vi "AllThingsBaxter_ROS.vi"   [LabVIEW 2012]
uses:
  <userlib>/ROSforLV/ROS/MessageBuilding/std_msgs/subs/boolScalar.vi
  <userlib>/ROSforLV/ROS/MessageBuilding/std_msgs/subs/durationScalar.vi
  <userlib>/ROSforLV/ROS/MessageBuilding/std_msgs/subs/float32Scalar.vi
  <userlib>/ROSforLV/ROS/MessageBuilding/std_msgs/subs/float64Scalar.vi
  <userlib>/ROSforLV/ROS/MessageBuilding/std_msgs/subs/i8Scalar.vi
  <userlib>/ROSforLV/ROS/MessageBuilding/std_msgs/subs/i16Scalar.vi
  <userlib>/ROSforLV/ROS/MessageBuilding/std_msgs/subs/i32Scalar.vi
  <userlib>/ROSforLV/ROS/MessageBuilding/std_msgs/subs/i64Scalar.vi
  <userlib>/ROSforLV/ROS/MessageBuilding/std_msgs/subs/stringScalar.vi
  <userlib>/ROSforLV/ROS/MessageBuilding/std_msgs/subs/timeScalar.vi
  <userlib>/ROSforLV/ROS/MessageBuilding/std_msgs/subs/u8Scalar.vi
  <userlib>/ROSforLV/ROS/MessageBuilding/std_msgs/subs/u16Scalar.vi
  <userlib>/ROSforLV/ROS/MessageBuilding/std_msgs/subs/u32Scalar.vi
  <userlib>/ROSforLV/ROS/MessageBuilding/std_msgs/subs/u64Scalar.vi
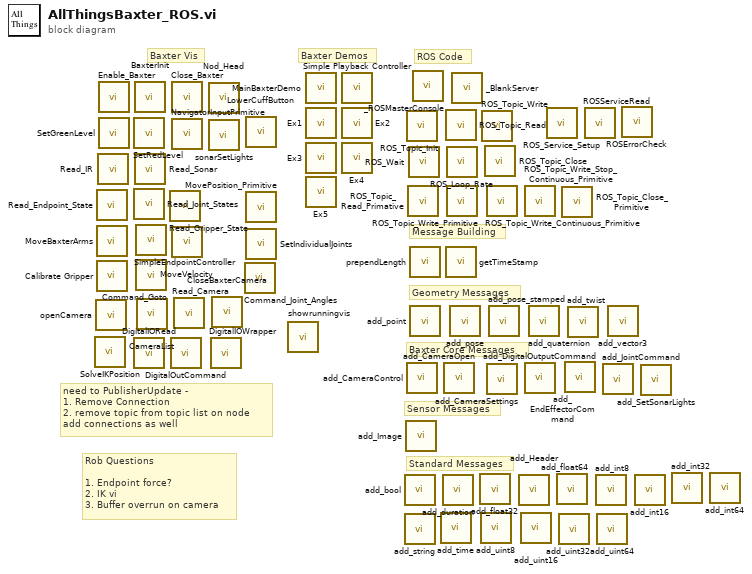
[diagram p0: block diagram]
diagram:
  # "Standard Messages"
  # "Sensor Messages"
  # "Baxter Core Messages"
  # "Geometry Messages"
  # "Message Building"
  # "Rob Questions\n\n1. Endpoint force?\n2. IK vi\n3. Buffer overrun on camera"
  # "need to PublisherUpdate - \n1. Remove Connection\n2. remove topic from topic list on node\nadd connections as well"
  # "ROS Code"
  # "Baxter Demos"
  # "Baxter Vis"
  n1 = call <userlib>:"SolveIKPosition.vi"() -> ()  [unwired: 7 in, 1 out]
  n2 = call <userlib>:"openCamera.vi"() -> ()  [unwired: 3 in, 2 out]
  n3 = call <userlib>:"Read_Endpoint_State.vi"() -> ()  [unwired: 3 in, 2 out]
  n4 = call <userlib>:"MoveBaxterArms.vi"() -> ()  [unwired: 6 in, 1 out]
  n5 = call <userlib>:"Calibrate Gripper.vi"() -> ()  [unwired: 6 in, 1 out]
  n6 = call <userlib>:"Read_IR.vi"() -> ()  [unwired: 3 in, 2 out]
  n7 = call <userlib>:"Enable_Baxter.vi"() -> ()  [unwired: 4 in, 1 out]
  n8 = call <userlib>:"SetGreenLevel.vi"() -> ()  [unwired: 3 in, 1 out]
  n9 = call <userlib>:"SetRedLevel.vi"() -> ()  [unwired: 3 in, 1 out]
  n10 = call <userlib>:"Read_Joint_States.vi"() -> ()  [unwired: 3 in, 2 out]
  n11 = call <userlib>:"DigitalIORead.vi"() -> ()  [unwired: 4 in, 2 out]
  n12 = call <userlib>:"BaxterInit.vi"() -> ()  [unwired: 12 in]
  n13 = call <userlib>:"Read_Sonar.vi"() -> ()  [unwired: 3 in, 2 out]
  n14 = call <userlib>:"SimpleEndpointController.vi"() -> ()  [unwired: 5 in, 1 out]
  n15 = call <userlib>:"Command_Goto.vi"() -> ()  [unwired: 6 in, 1 out]
  n16 = call <userlib>:"CameraList.vi"() -> ()  [unwired: 2 in, 2 out]
  n17 = call <userlib>:"Read_Gripper_State.vi"() -> ()  [unwired: 3 in, 2 out]
  n18 = call <userlib>:"DigitalOutCommand.vi"() -> ()  [unwired: 5 in, 1 out]
  n19 = call <userlib>:"Close_Baxter.vi"() -> ()  [unwired: 4 in, 1 out]
  n20 = call <userlib>:"NavigatorInputPrimitive.vi"() -> ()  [unwired: 3 in, 2 out]
  n21 = call <userlib>:"MoveVelocity.vi"() -> ()  [unwired: 6 in, 1 out]
  n22 = call <userlib>:"Read_Camera.vi"() -> ()  [unwired: 3 in, 2 out]
  n23 = call <userlib>:"Nod_Head.vi"() -> ()  [unwired: 4 in, 1 out]
  n24 = call <userlib>:"sonarSetLights.vi"() -> ()  [unwired: 4 in, 1 out]
  n25 = call <userlib>:"DigitalIOWrapper.vi"() -> ()  [unwired: 3 in, 2 out]
  n26 = call <userlib>:"CloseBaxterCamera.vi"() -> ()  [unwired: 3 in, 3 out]
  n27 = call <userlib>:"Command_Joint_Angles.vi"() -> ()  [unwired: 6 in, 1 out]
  n28 = call <userlib>:"LowerCuffButton.vi"() -> ()  [unwired: 3 in, 2 out]
  n29 = call <userlib>:"MovePosition_Primitive.vi"() -> ()  [unwired: 6 in, 1 out]
  n30 = call <userlib>:"SetIndividualJoints.vi"() -> ()  [unwired: 6 in, 1 out]
  n31 = call <userlib>:"showrunningvis.vi"() -> ()  [unwired: 1 in]
  n32 = call <userlib>:"MainBaxterDemo.vi"() -> ()  [unwired: 12 in]
  n33 = call <userlib>:"Ex1.vi"() -> ()  [unwired: 12 in]
  n34 = call <userlib>:"Ex3.vi"() -> ()  [unwired: 12 in]
  n35 = call <userlib>:"Ex5.vi"() -> ()  [unwired: 12 in]
  n36 = call <userlib>:"Simple Playback Controller.vi"() -> ()  [unwired: 12 in]
  n37 = call <userlib>:"Ex2.vi"() -> ()  [unwired: 12 in]
  n38 = call <userlib>:"Ex4.vi"() -> ()  [unwired: 12 in]
  n39 = call-poly <userlib>:"add_bool.vi"() -> ()  [unwired: 5 in, 1 out]
  n40 = call-poly <userlib>:"add_string.vi"() -> ()  [unwired: 5 in, 1 out]
  n41 = call <userlib>:"add_Image.vi"() -> ()  [unwired: 5 in, 1 out]
  n42 = call <userlib>:"ROS_Topic_Init.vi"() -> ()  [unwired: 3 in, 1 out]
  n43 = call <userlib>:"add_CameraControl.vi"() -> ()  [unwired: 5 in, 1 out]
  n44 = call <userlib>:"ROS_Topic_Read_Primative.vi"() -> ()  [unwired: 2 in, 2 out]
  n45 = call <userlib>:"ROS_Wait.vi"() -> ()  [unwired: 6 in, 1 out]
  n46 = call <userlib>:"prependLength.vi"() -> ()  [unwired: 5 in, 1 out]
  n47 = call <userlib>:"add_point.vi"() -> ()  [unwired: 5 in, 1 out]
  n48 = call <userlib>:"_ROSMasterConsole.vi"() -> ()  [unwired: 12 in]
  n49 = call-poly <userlib>:"add_time.vi"() -> ()  [unwired: 5 in, 1 out]
  n50 = call-poly <userlib>:"add_duration.vi"() -> ()  [unwired: 5 in, 1 out]
  n51 = call <userlib>:"add_CameraOpen.vi"() -> ()  [unwired: 5 in, 1 out]
  n52 = call <userlib>:"ROS_Topic_Read.vi"() -> ()  [unwired: 2 in, 2 out]
  n53 = call <userlib>:"getTimeStamp.vi"() -> ()  [unwired: 2 in, 3 out]
  n54 = call <userlib>:"ROS_Loop_Rate.vi"() -> ()  [unwired: 5 in, 2 out]
  n55 = call <userlib>:"ROS_Topic_Write_Primitive.vi"() -> ()  [unwired: 3 in, 1 out]
  n56 = call <userlib>:"add_pose.vi"() -> ()  [unwired: 5 in, 1 out]
  n57 = call <userlib>:"_BlankServer.vi"() -> ()  [unwired: 4 in]
  n58 = call-poly <userlib>:"add_float32.vi"() -> ()  [unwired: 5 in, 1 out]
  n59 = call-poly <userlib>:"add_uint8.vi"() -> ()  [unwired: 5 in, 1 out]
  n60 = call <userlib>:"ROS_Topic_Write.vi"() -> ()  [unwired: 4 in, 1 out]
  n61 = call <userlib>:"ROS_Topic_Close.vi"() -> ()  [unwired: 4 in, 1 out]
  n62 = call <userlib>:"ROS_Topic_Write_Continuous_Primitive.vi"() -> ()  [unwired: 3 in, 1 out]
  n63 = call <userlib>:"add_CameraSettings.vi"() -> ()  [unwired: 5 in, 1 out]
  n64 = call <userlib>:"add_pose_stamped.vi"() -> ()  [unwired: 5 in, 1 out]
  n65 = call <userlib>:"add_Header.vi"() -> ()  [unwired: 5 in, 1 out]
  n66 = call-poly <userlib>:"add_uint16.vi"() -> ()  [unwired: 5 in, 1 out]
  n67 = call <userlib>:"ROS_Topic_Write_Stop_Continuous_Primitive.vi"() -> ()  [unwired: 3 in, 1 out]
  n68 = call <userlib>:"add_DigitalOutputCommand.vi"() -> ()  [unwired: 5 in, 1 out]
  n69 = call <userlib>:"add_quaternion.vi"() -> ()  [unwired: 5 in, 1 out]
  n70 = call <userlib>:"ROS_Service_Setup.vi"() -> ()  [unwired: 5 in, 3 out]
  n71 = call-poly <userlib>:"add_float64.vi"() -> ()  [unwired: 5 in, 1 out]
  n72 = call-poly <userlib>:"add_uint32.vi"() -> ()  [unwired: 5 in, 1 out]
  n73 = call <userlib>:"ROS_Topic_Close_Primitive.vi"() -> ()  [unwired: 3 in, 1 out]
  n74 = call <userlib>:"add_EndEffectorCommand.vi"() -> ()  [unwired: 5 in, 1 out]
  n75 = call <userlib>:"add_twist.vi"() -> ()  [unwired: 5 in, 1 out]
  n76 = call <userlib>:"ROSServiceRead.vi"() -> ()  [unwired: 2 in, 3 out]
  n77 = call-poly <userlib>:"add_int8.vi"() -> ()  [unwired: 5 in, 1 out]
  n78 = call-poly <userlib>:"add_uint64.vi"() -> ()  [unwired: 5 in, 1 out]
  n79 = call <userlib>:"add_JointCommand.vi"() -> ()  [unwired: 11 in, 1 out]
  n80 = call <userlib>:"add_vector3.vi"() -> ()  [unwired: 5 in, 1 out]
  n81 = call <userlib>:"ROSErrorCheck.vi"() -> ()  [unwired: 3 in, 1 out]
  n82 = call-poly <userlib>:"add_int16.vi"() -> ()  [unwired: 5 in, 1 out]
  n83 = call <userlib>:"add_SetSonarLights.vi"() -> ()  [unwired: 5 in, 1 out]
  n84 = call-poly <userlib>:"add_int32.vi"() -> ()  [unwired: 5 in, 1 out]
  n85 = call-poly <userlib>:"add_int64.vi"() -> ()  [unwired: 5 in, 1 out]
